vi "xijk_remove_cluster_filenames.vi"(8 "error in":errorcluster, 11 "filepaths in":T2) -> (0 "error out":errorcluster, 3 "filenames out":T1)   [LabVIEW 2010]
uses:
  Type Def/filepath.ctl
  Type Def/indicator_filepaths.ctl
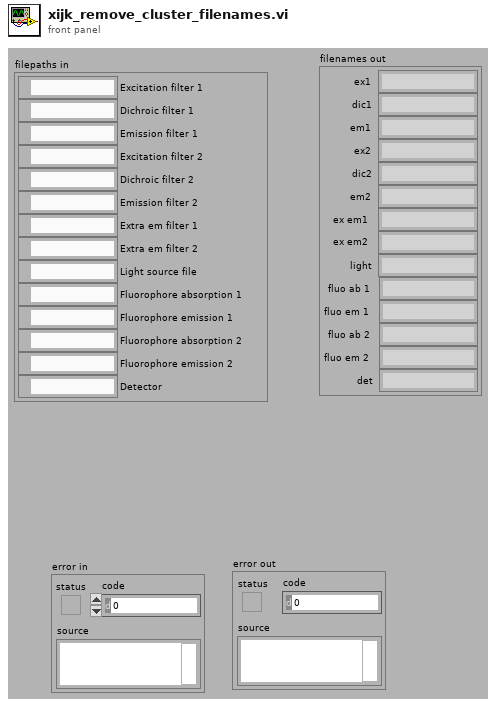
[diagram p1: front panel]
types:
  T1 = typedef "indicator_filepaths.ctl" = cluster{"ex1":string, "dic1":string, "em1":string, "ex2":string, "dic2":string, "em2":string, "ex em1":string, "ex em2":string, "light":string, "fluo ab 1":string, "fluo em 1":string, "fluo ab 2":string, "fluo em 2":string, "det":string}
  T2 = typedef "filepath.ctl" = cluster{"Excitation filter 1":path, "Dichroic filter 1":path, "Emission filter 1":path, "Excitation filter 2":path, "Dichroic filter 2":path, "Emission filter 2":path, "Extra em filter 1":path, "Extra em filter 2":path, "Light source file":path, "Fluorophore absorption 1":path, "Fluorophore emission 1":path, "Fluorophore absorption 2":path, "Fluorophore emission 2":path, "Detector":path}
  T3 = cluster{"[0]":string, "[1]":string, "[2]":string, "[3]":string, "[4]":string, "[5]":string, "[6]":string, "[7]":string, "[8]":string, "[9]":string, "[10]":string, "[11]":string, "[12]":string, "[13]":string}
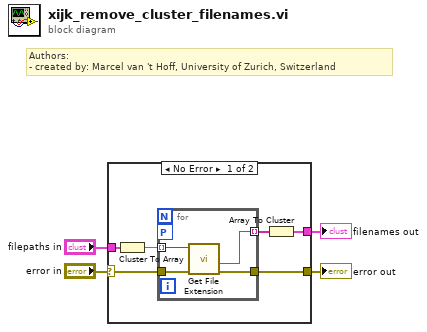
[diagram p0: block diagram]
diagram:
  # "Authors: \n- created by: Marcel van 't Hoff, University of Zurich, Switzerland"
  n1 = case shown="No Error" "error in" {
    selector: "error in" -> [w6 w15]
    tunnel: "filepaths in" -> [w7 _]
    tunnel: [w8 _] -> w3
    tunnel: [w5 w15] -> w1
    frame No Error {
      n2 = Cluster To Array(cluster=w7) -> (array=w10:path[])
      n3 = for {
        tunnel: [w13] -> w9 mode=indexing
        tunnel: w10 -> [w14] mode=indexing
        workers-P: _ -> [_]
        tunnel: w6 -> [w12]
        tunnel: [w11] -> w5
        n4 = call <vilib>:"Get File Extension.vi"("error in (no error)"=w12, "file"=w14) -> ("error out"=w11:errorcluster, "filename without extension"=w13:string)  [unwired: 6 in, 2 out]
      }
      n5 = Array To Cluster(array=w9) -> (cluster=w8:T3)
    }
    frame Error {
    }
  }
  "error out" <- w1
  "filenames out" <- w3
